vi "monstera_deliciosa_hygro&termometer.vi"() -> ()   [LabVIEW 2020]
uses:
  <vilib>/Instr/_visa.llb/VISA Configure Serial Port (Instr).vi
panel:
  out "Increase":bool
  out "Decrease":bool
  out "Temperature":i32(graph)
  out "Humidity":i32(graph)
  out "Heater":bool
  out "Cooler":bool
  out "Hygrometer":i32(slide) scale=0.0..100.0
  out "SENT":bool=TRUE
  out "temp":string
  out "hum":string
  in  "Date/Time e mail":timestamp
  out "Real Time":timestamp
  out "Thermometer":i32(slide) scale=0.0..100.0
  out "Humidity":i32
  in  "STOP":bool
  out "Temperature":i32
  in  "Serial Port":refnum<visa-resource-name>
  # "MONSTERA DELICIOSA'S AUTOMATION \nWITH HYGROMETER AND THERMOMETER"
  # "TEMPERATURE"
  # "HUMIDITY"
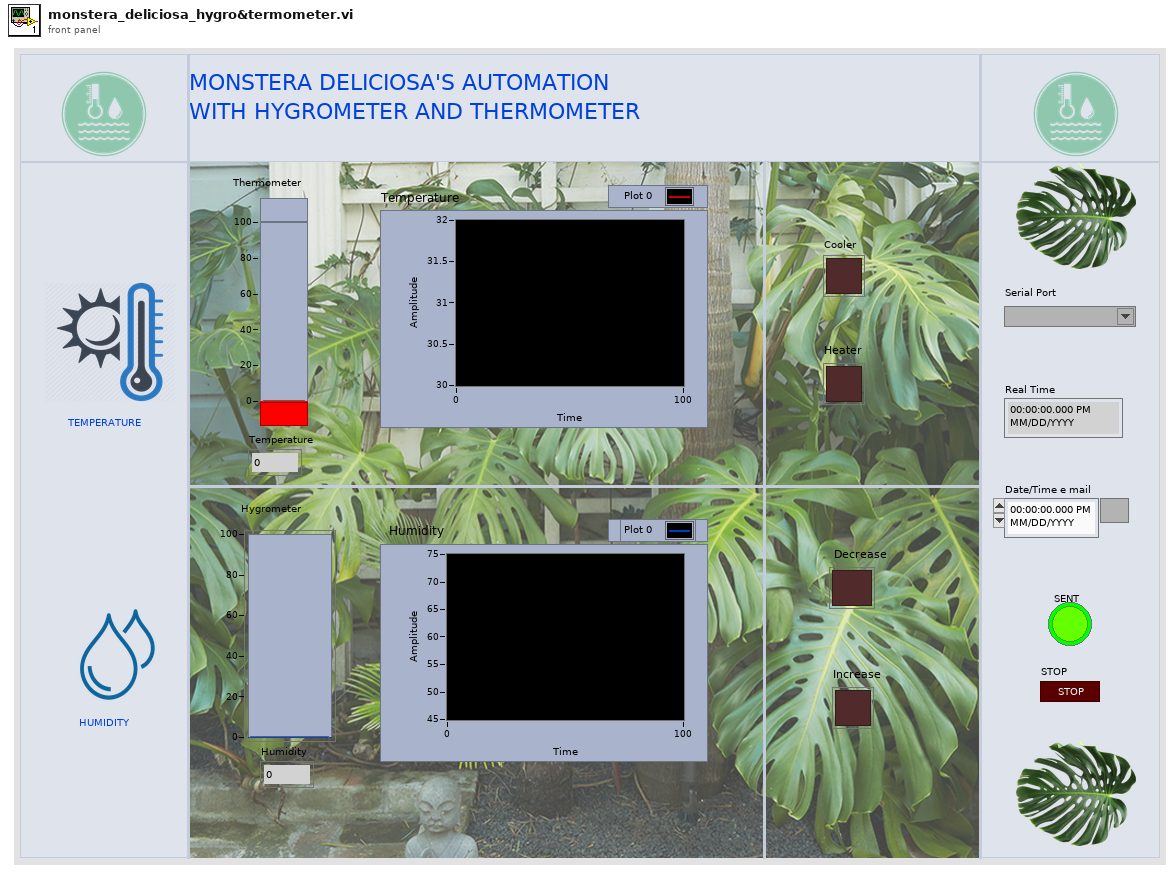
[diagram p1: front panel]
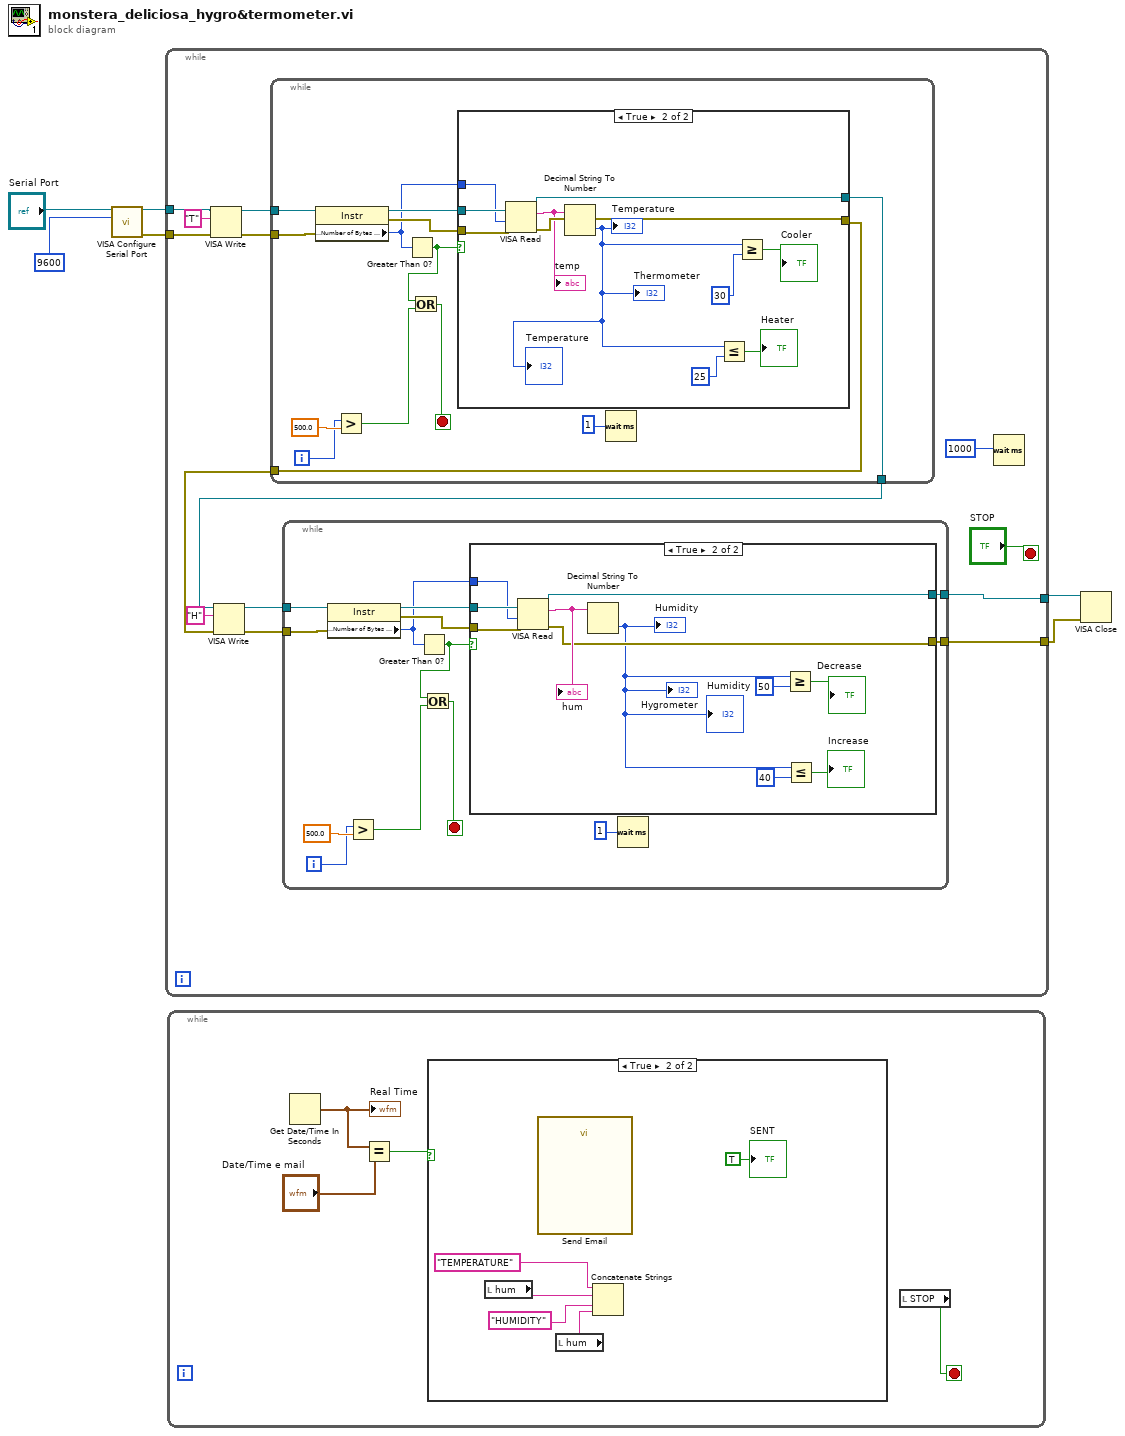
[diagram p0: block diagram]
diagram:
  n1 = call-poly "VISA Configure Serial Port"("VISA resource name"="Serial Port", "baud rate (9600)"=u32 9600) -> ("VISA resource name out"=w4:refnum<visa-resource-name>, "error out"=w3:errorcluster)  [unwired: 12 in]
  n2 = while {
    tunnel: w4 -> [w20]
    tunnel: w3 -> [w19]
    tunnel: [w8] -> w2
    tunnel: [w7] -> w1
    stop <- "STOP" stop-if-true
    n3 = VISA Write(VISA resource name=w20, write buffer="T", error in (no error)=w19) -> (VISA resource name out=w17:refnum<visa-resource-name>, error out=w16:errorcluster)  [unwired: 1 out]
    n4 = while {
      tunnel: w17 -> [w59]
      tunnel: w16 -> [w58]
      tunnel: [w48] -> w10
      tunnel: [w47] -> w9
      i -> [w52]
      stop <- w49 stop-if-true
      n5 = property class="Instr"(reference=w59, error in=w58) -> (reference out=w57:refnum<visa-resource-name>, error out=w56:errorcluster, "Serial Settings:Number of Bytes at Serial Port"=w55:u32)
      n6 = Greater?(x=w52, y=500.0) -> (0:w50:bool)
      n7 = Greater Than 0?(x=w55) -> (x > 0?=w51:bool)
      n8 = Or(x=w51, y=w50) -> (x .or. y?=w49:bool)
      n9 = case shown="True" w51 {
        tunnel: w57 -> [w61 w72]
        tunnel: w56 -> [w60 w71]
        tunnel: w55 -> [_ w70]
        tunnel: [w61 w69] -> w48
        tunnel: [w60 w68] -> w47
        frame False {
        }
        frame True {
          n10 = VISA Read(VISA resource name=w72, byte count=w70, error in (no error)=w71) -> (VISA resource name out=w69:refnum<visa-resource-name>, read buffer=w67:string, error out=w68:errorcluster)  [unwired: 1 out]
          "temp" <- w67
          n11 = Decimal String To Number(string=w67) -> (number=w62:i32)  [unwired: 2 in, 1 out]
          "Temperature" <- w62
          "Thermometer" <- w62
          "Temperature" <- w62
          n12 = Less Or Equal?(x=w62, y=25) -> (x <= y?=→"Heater":bool)
          n13 = Greater Or Equal?(x=w62, y=30) -> (x >= y?=→"Cooler":bool)
        }
      }
      n14 = Wait (ms)(milliseconds to wait=u32 1 ("millisecond timer value")) -> ()  [unwired: 1 out]
    }
    n15 = VISA Write(VISA resource name=w10, write buffer="H", error in (no error)=w9) -> (VISA resource name out=w12:refnum<visa-resource-name>, error out=w11:errorcluster)  [unwired: 1 out]
    n16 = while {
      tunnel: w12 -> [w33]
      tunnel: w11 -> [w32]
      tunnel: [w28] -> w8
      tunnel: [w27] -> w7
      i -> [w24]
      stop <- w21 stop-if-true
      n17 = property class="Instr"(reference=w33, error in=w32) -> (reference out=w31:refnum<visa-resource-name>, error out=w30:errorcluster, "Serial Settings:Number of Bytes at Serial Port"=w29:u32)
      n18 = Greater?(x=w24, y=500.0) -> (0:w22:bool)
      n19 = Greater Than 0?(x=w29) -> (x > 0?=w23:bool)
      n20 = Or(x=w23, y=w22) -> (x .or. y?=w21:bool)
      n21 = case shown="True" w23 {
        tunnel: w31 -> [w35 w46]
        tunnel: w30 -> [w34 w45]
        tunnel: w29 -> [_ w44]
        tunnel: [w35 w42] -> w28
        tunnel: [w34 w41] -> w27
        frame False {
        }
        frame True {
          n22 = VISA Read(VISA resource name=w46, byte count=w44, error in (no error)=w45) -> (VISA resource name out=w42:refnum<visa-resource-name>, read buffer=w43:string, error out=w41:errorcluster)  [unwired: 1 out]
          "hum" <- w43
          n23 = Decimal String To Number(string=w43) -> (number=w38:i32)  [unwired: 2 in, 1 out]
          "Humidity" <- w38
          "Hygrometer" <- w38
          "Humidity" <- w38
          n24 = Greater Or Equal?(x=w38, y=50) -> (x >= y?=→"Decrease":bool)
          n25 = Less Or Equal?(x=w38, y=40) -> (x <= y?=→"Increase":bool)
        }
      }
      n26 = Wait (ms)(milliseconds to wait=u32 1 ("millisecond timer value")) -> ()  [unwired: 1 out]
    }
    n27 = Wait (ms)(milliseconds to wait=u32 1000 ("millisecond timer value")) -> ()  [unwired: 1 out]
  }
  n28 = while {
    stop <- w73 stop-if-true
    n29 = Get Date/Time In Seconds() -> (seconds since 1Jan1904=w76:timestamp)
    "Real Time" <- w76
    n30 = Equal?(x=w76, y="Date/Time e mail") -> (x = y?=w74:bool)
    n31 = case shown="True" w74 {
      frame False {
      }
      frame True {
        n32 = local read "hum"() -> (w78:string)
        n33 = call "Send Email"() -> ()  [unwired: 11 in, 1 out]
        n34 = local read "hum"() -> (w79:string)
        n35 = Concatenate Strings("TEMPERATURE" ("string"), w78, "HUMIDITY" ("string"), w79) -> ()  [unwired: 1 out]
        "SENT" <- TRUE
      }
    }
    n36 = local read "STOP"() -> (w73:bool)
  }
  n37 = VISA Close(VISA resource name=w2, error in (no error)=w1) -> ()  [unwired: 1 out]
